vi "Open RFmx.vi"(8 "error in":errorcluster {"code" format="%.0x"}, 10 "Bitfile":string="niVSTFPGA_UART.lvbitx", 11 "resource name":refnum<k15>) -> (0 "error out":errorcluster {"code" format="%.0x"}, 3 "Instrument Handle Out":refnum<k21>)   [LabVIEW 2018]
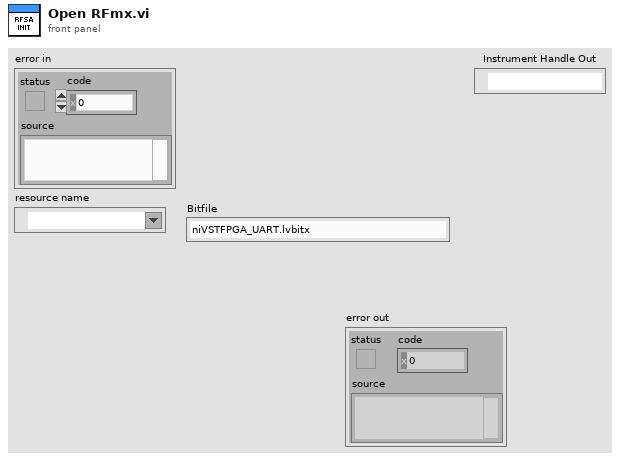
[diagram p1: front panel]
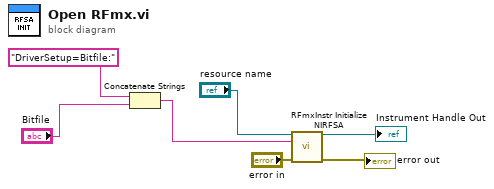
[diagram p0: block diagram]
diagram:
  n1 = Concatenate Strings("DriverSetup=Bitfile:" ("string"), "Bitfile") -> (w4:string)
  n2 = call <vilib>:"RFmxInstr Initialize NIRFSA.vi"("Resource Name"="resource name", "Option String"=w4, "error in (no error)"="error in") -> ("Instrument Handle Out"=→"Instrument Handle Out":refnum<k21>, "error out"=→"error out":errorcluster)  [unwired: 10 in, 1 out]
